vi "Ej 3.2.vi"() -> ()   [LabVIEW 2013]
uses:
  <vilib>/sound2/lvsound2.llb/Sound Output Write (DBL Single).vi
panel:
  in  "Cluster":T1={"Sample rate (S/s)"=1000.0, "Number of channels"=2, "bits per sample"=16}
  out "Triangle":dbl[](graph)
  out "Rampa":dbl[](graph)
  out "Cuadrada":dbl[](graph)
  in  "Stop Button":bool
  out "Senoidal":dbl[](graph)
  in  "Amplitud":i32=1
  in  "Frecuencia":dbl=50.0
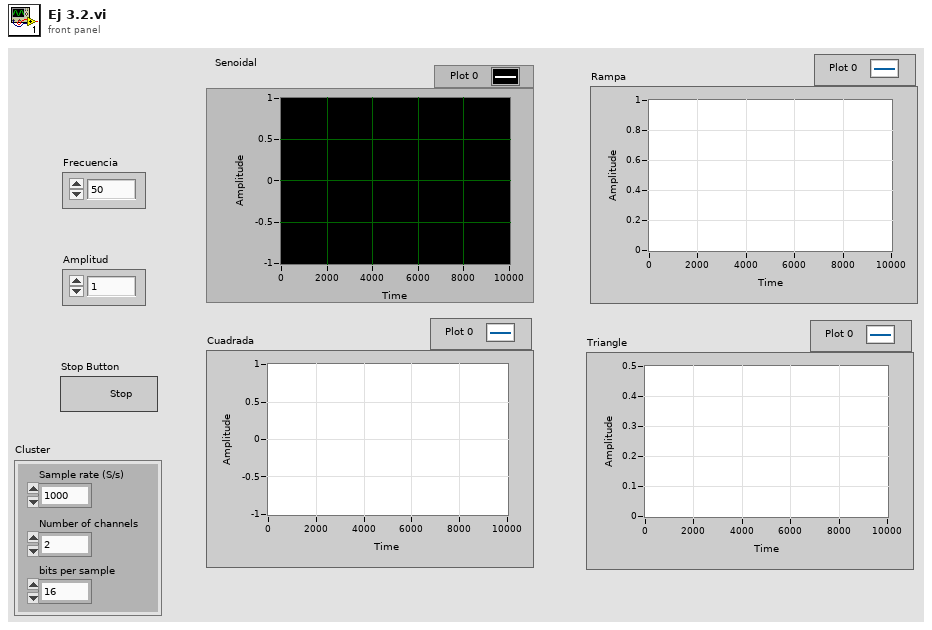
[diagram p1: front panel]
types:
  T1 = cluster{"Sample rate (S/s)":dbl, "Number of channels":i32, "bits per sample":i32}
  T2 = typedef "Sound Output Task ID.ctl" = u32
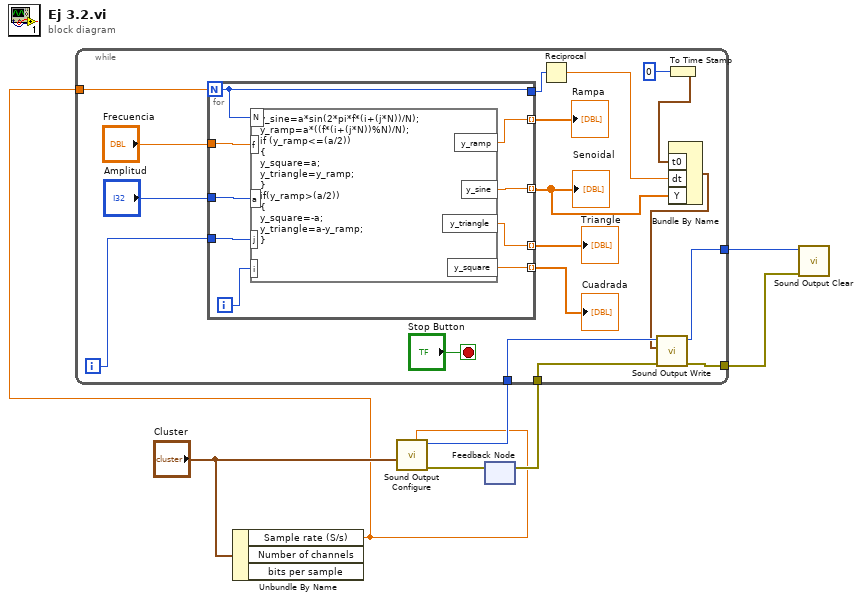
[diagram p0: block diagram]
diagram:
  n1 = Unbundle By Name("Cluster") -> ("Sample rate (S/s)"=w1:dbl)  [unwired: 2 out]
  n2 = call <vilib>:"Sound Output Configure.vi"("number of samples/ch"=w1, "sound format"="Cluster") -> ("error out"=w6:errorcluster, "task ID"=w2:T2)  [unwired: 8 in]
  n3 = feedback-in #1(w6) -> ()
  n4 = feedback #1() -> (w5:errorcluster)  [unwired: 1 in]
  n5 = while {
    tunnel: w1 -> [w19]
    tunnel: w5 -> [w18]
    tunnel: [w17] -> w4
    tunnel: [w12] -> w3
    tunnel: w2 -> [w11]
    i -> [w24]
    stop <- "Stop Button" stop-if-true
    n6 = for {
      N: w19 -> [w26]
      tunnel: "Frecuencia" -> [w34]
      tunnel: "Amplitud" -> [w33]
      tunnel: [w32] -> w15 mode=indexing
      tunnel: w24 -> [w30]
      tunnel: [w29] -> w21 mode=indexing
      tunnel: [w28] -> w16 mode=indexing
      tunnel: [w27] -> w20 mode=indexing
      tunnel: [w26] -> w14
      i -> [w31]
      n7 = formula code="y_sine=a*sin(2*pi*f*(i+(j*N))/N);\ny_ramp=a*((f*(i+(j*N))%N)/N);\nif (y_ramp<=(a/2))\n{\ny_square=a;\ny_triangle=y_ramp;\n}\nif(y_ramp>(a/2))\n{\ny_square=-a;\ny_triangle=a-y_ramp;\n}"("f"=w34, "a"=w33, "N"=w26, "i"=w31, "j"=w30) -> ("y_sine"=w32:dbl, "y_square"=w29:dbl, "y_ramp"=w28:dbl, "y_triangle"=w27:dbl)
    }
    "Senoidal" <- w15
    "Cuadrada" <- w21
    "Rampa" <- w16
    "Triangle" <- w20
    n8 = Reciprocal(x=w14) -> (1/x=w13:dbl)
    n9 = To Time Stamp(1:0) -> (0:w10:timestamp)
    n10 = Bundle By Name("t0"=w10, "dt"=w13, "Y"=w15) -> (w8:waveform(dbl))  [unwired: 1 in]
    n11 = call-poly <vilib>:"Sound Output Write.vi"("error in (no error)"=w18, "data"=w8, "task ID"=w11) -> ("error out"=w17:errorcluster, "task ID out"=w12:T2)  [unwired: 7 in]
  }
  n12 = call <vilib>:"Sound Output Clear.vi"("error in (no error)"=w4, "task ID"=w3) -> ()  [unwired: 9 in, 1 out]
